vi "Set Start Sequence Button LED.vi"(4 "error in":errorcluster, 6 "Start LED":bool) -> (0 "error out":errorcluster)   [LabVIEW 2015]
uses:
  <vilib>/DAQmx/write.llb/DAQmx Write (Digital Bool 1Line 1Point).vi
  <vilib>/DAQmx/miscellaneous.llb/DAQmx Fill In Error Info.vi
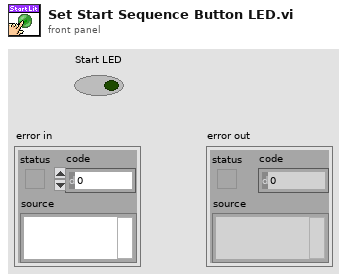
[diagram p1: front panel]
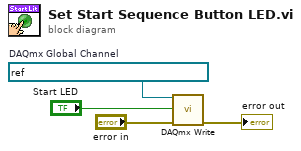
[diagram p0: block diagram]
diagram:
  w4 = refnum<k21> "DO13 Start Sequence Button LED"  # DAQmx Global Channel
  n1 = call-poly <vilib>:"DAQmx Write.vi"("task/channels in"=w4, "data"="Start LED", "error in"="error in") -> ("error out"=→"error out":errorcluster)  [unwired: 10 in, 2 out]
